vi "etlUSBOpen.vi"(0 "lens":enum16{"0", "1"}(ring)) -> (1 "read buffer":string)   [LabVIEW 2017]
uses:
  globalDevices.vi
  <vilib>/Instr/_visa.llb/VISA Configure Serial Port (Instr).vi
panel:
  out "return count 2":u32
  out "return count":u32
  out "read buffer 2":string
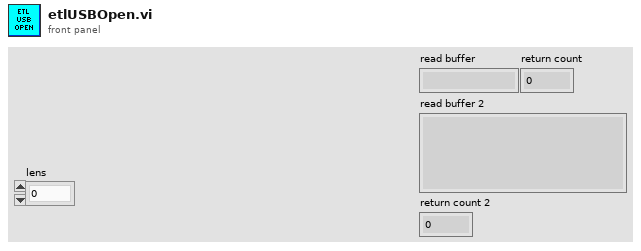
[diagram p1: front panel]
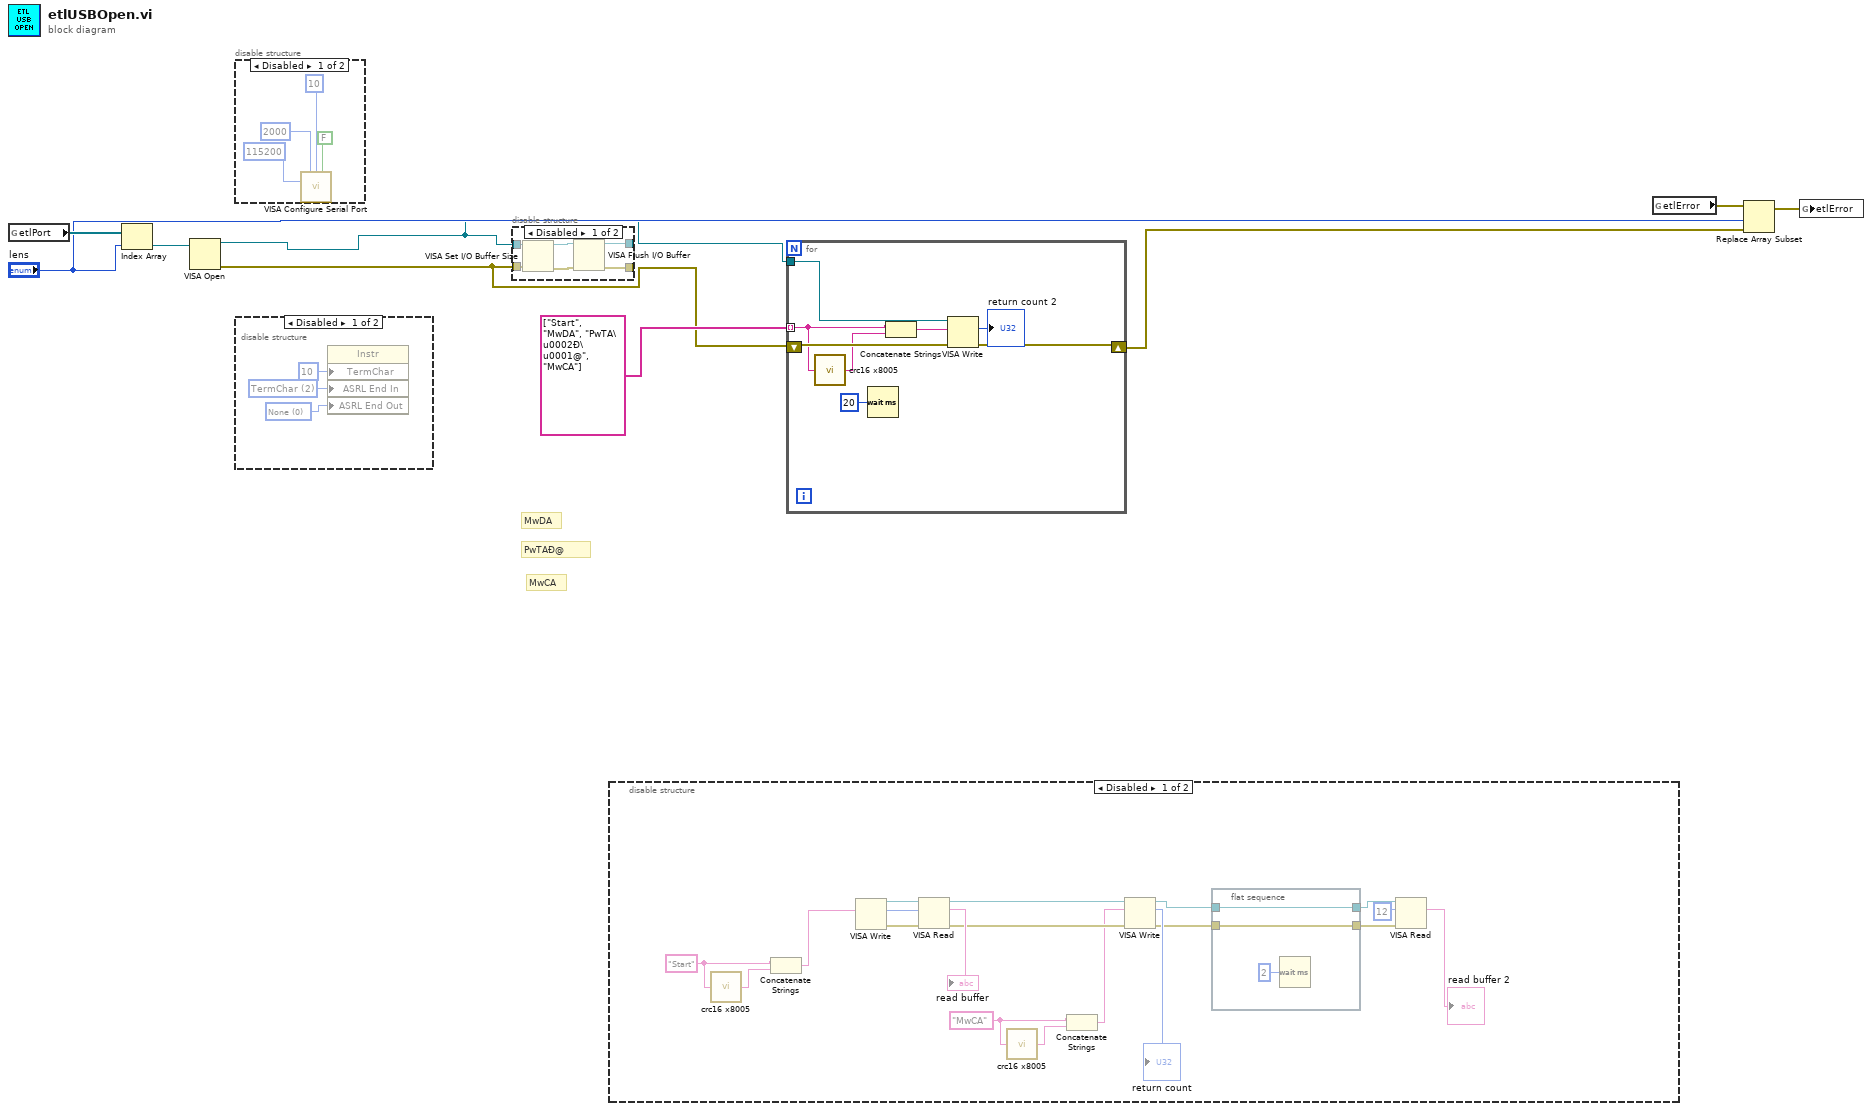
[diagram p0: block diagram]
diagram:
  # "MwCA"
  # "MwDA"
  # "PwTAÐ@"
  n1 = global read "globalDevices.vi" "etlPort"() -> (w9:refnum<visa-resource-name>[])
  n2 = Index Array(array=w9, index="lens") -> (element=w8:refnum<visa-resource-name>)
  n3 = VISA Open(VISA resource name=w8) -> (VISA resource name=w2:refnum<visa-resource-name>, error out=w1:errorcluster)  [unwired: 4 in]
  n4 = disable-structure shown="Disabled" {
    frame Disabled {
      n5 = call-poly "VISA Configure Serial Port"("timeout (10sec)"=u32 2000, "termination char\n(0xA = '\\n' = LF)"=u8 10 ("termination char\n(0xA = '\\n' = LF)"), "Enable Termination\nChar (T)"=FALSE ("Enable Termination\nChar (T)"), "baud rate (9600)"=u32 115200) -> ()  [unwired: 10 in, 2 out]
    }
    frame Enabled {
    }
  }
  n6 = disable-structure shown="Disabled" {
    frame Disabled {
      w15 = u16 0 items=["None", "Last Bit", "TermChar", "Break"] ("Serial Settings:End Mode for Writes")
      w16 = u16 2 items=["None", "Last Bit", "TermChar"] ("Serial Settings:End Mode for Reads")
      n7 = property class="Instr"("TermChar"=u8 10 ("Message Based Settings:Termination Character"), "ASRL End In"=w16, "ASRL End Out"=w15) -> ()  [unwired: 2 in, 2 out]
    }
    frame Enabled {
    }
  }
  n8 = disable-structure shown="Disabled" {
    disable-tunnel: [w20 _] -> _
    disable-tunnel: [w19 _] -> _
    disable-tunnel: w2 -> [w18 _]
    disable-tunnel: w1 -> [w17 _]
    frame Disabled {
      n9 = VISA Set I/O Buffer Size(VISA resource name=w18, error in (no error)=w17) -> (VISA resource name out=w22:refnum<visa-resource-name>, error out=w21:errorcluster)  [unwired: 2 in]
      n10 = VISA Flush I/O Buffer(VISA resource name=w22, error in (no error)=w21) -> (VISA resource name out=w20:refnum<visa-resource-name>, error out=w19:errorcluster)  [unwired: 1 in]
    }
    frame Enabled {
    }
  }
  n11 = disable-structure shown="Disabled" {
    frame Disabled {
      w32 = "MwCA" ("write buffer")
      w36 = "Start" ("write buffer")
      n12 = call "crc16 x8005.vi"("message"=w36) -> ("CRC16"=w37:string)  [unwired: 4 in]
      n13 = Concatenate Strings(w36, w37) -> (w35:string)
      n14 = VISA Write(write buffer=w35) -> (VISA resource name out=w41:refnum<visa-resource-name>, return count=w40:u32, error out=w39:errorcluster)  [unwired: 2 in]
      n15 = VISA Read(VISA resource name=w41, byte count=w40, error in (no error)=w39) -> (VISA resource name out=w33:refnum<visa-resource-name>, read buffer=→"read buffer":string, error out=w34:errorcluster)  [unwired: 1 out]
      n16 = call "crc16 x8005.vi"("message"=w32) -> ("CRC16"=w31:string)  [unwired: 4 in]
      n17 = Concatenate Strings(w32, w31) -> (w30:string)
      n18 = VISA Write(VISA resource name=w33, write buffer=w30, error in (no error)=w34) -> (VISA resource name out=w26:refnum<visa-resource-name>, return count=→"return count":u32, error out=w24:errorcluster)
      n19 = flat-sequence {
        tunnel: w26 -> [w43]
        tunnel: [w43] -> w25
        tunnel: w24 -> [w42]
        tunnel: [w42] -> w23
        frame #0 {
          n20 = Wait (ms)(milliseconds to wait=u32 2) -> ()  [unwired: 1 out]
        }
      }
      n21 = VISA Read(VISA resource name=w25, byte count=u32 12, error in (no error)=w23) -> (read buffer=→"read buffer 2":string)  [unwired: 3 out]
    }
    frame Enabled {
    }
  }
  n22 = for {
    tunnel: string[] ["Start", "MwDA", "PwTA\u0002Ð\u0001@", "MwCA"] -> [w48] mode=indexing
    tunnel: w2 -> [w52]
    shift-right: [w50] -> w3
    shift-left: w1 -> [w49]
    n23 = call "crc16 x8005.vi"("message"=w48) -> ("CRC16"=w47:string)  [unwired: 4 in]
    n24 = Wait (ms)(milliseconds to wait=u32 20) -> ()  [unwired: 1 out]
    n25 = Concatenate Strings(w48, w47) -> (w46:string)
    n26 = VISA Write(VISA resource name=w52, write buffer=w46, error in (no error)=w49) -> (return count=→"return count 2":u32, error out=w50:errorcluster)  [unwired: 1 out]
  }
  n27 = global read "globalDevices.vi" "etlError"() -> (w7:errorcluster[])
  n28 = Replace Array Subset(array=w7, new element=w3, index="lens") -> (w5:errorcluster[])
  n29 = global write "globalDevices.vi" "etlError"(w5) -> ()
